vi "ReportGenerator.Chapter.vi"(8 "error in (no error)":errorcluster, 9 "Font":T1, 10 "Chapter":string, 11 "NI_report in":refnum<class "NI_report.lvclass">) -> (0 "error out":errorcluster, 3 "NI_report out":refnum<class "NI_report.lvclass">)   [LabVIEW 2019, in "Tools.lvlib"]
uses:
  <vilib>/Utility/NIReport.llb/NI_report.lvclass
  <vilib>/Utility/NIReport.llb/Append Report Text (str wrap).vi
  Tools.lvlib
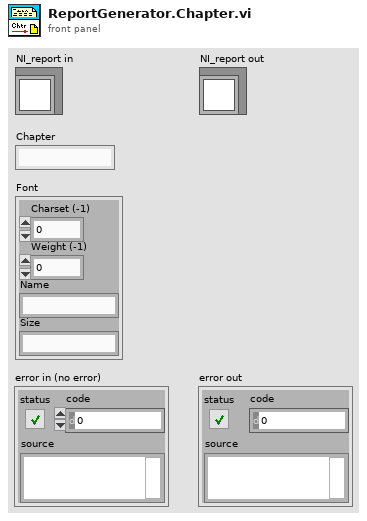
[diagram p1: front panel]
types:
  T1 = cluster{"Charset (-1)":i16, "Weight (-1)":i16, "Name":string, "Size":string}
  T2 = cluster{"Italic":enum16{"Italic Unchanged", "Italic On", "Italic Off"}, "Strike Through":enum16{"Strike Through Unchanged", "Strike Through On", "Strike Through Off"}, "Underline":enum16{"Underline Unchanged", "Underline On", "Underline Off"}, "Bold":enum16{"Bold Unchanged", "Bold On", "Bold Off"}}
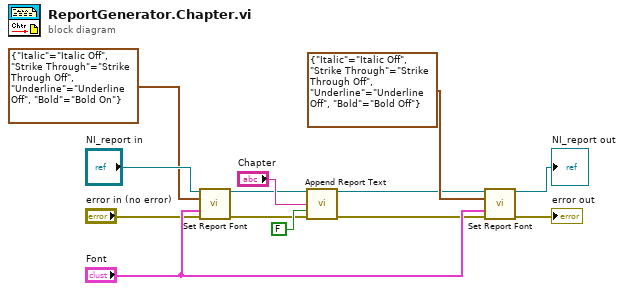
[diagram p0: block diagram]
diagram:
  n1 = call-dynamic "Set Report Font.vi"("report in"="NI_report in", "text options"=T2 {"Italic"=enum."Italic Off", "Strike Through"=enum."Strike Through Off", "Underline"=enum."Underline Off", "Bold"=enum."Bold On"}, "font settings"="Font", "error in (no error)"="error in (no error)") -> ("report out"=w4:refnum<class "NI_report.lvclass">, "error out"=w5:errorcluster)  [unwired: 9 in, 1 out]
  n2 = call-poly <vilib>:"Append Report Text.vi"("report in"=w4, "text"="Chapter", "append on new line? (F)"=FALSE, "error in (no error)"=w5) -> ("report out"=w2:refnum<class "NI_report.lvclass">, "error out"=w1:errorcluster)  [unwired: 8 in, 2 out]
  n3 = call-dynamic "Set Report Font.vi"("report in"=w2, "text options"=T2 {"Italic"=enum."Italic Off", "Strike Through"=enum."Strike Through Off", "Underline"=enum."Underline Off", "Bold"=enum."Bold Off"}, "font settings"="Font", "error in (no error)"=w1) -> ("report out"=→"NI_report out":refnum<class "NI_report.lvclass">, "error out"=→"error out":errorcluster)  [unwired: 9 in, 1 out]
